vi "Scaled Waveform.vi"(8 "Error In":errorcluster, 11 "Async State Vars In":T1) -> (0 "Error Out":errorcluster, 3 "Async State Vars Out":T1)   [LabVIEW 2015, in "Waveform-Processing-Custom-Device Shared.lvlib" / "Scaled Waveform.lvlib"]
uses:
  Shared/Scaled Waveform/Scaled Waveform.lvlib
  Types/AsyncStateVariables.ctl
  <vilib>/NI Veristand/Custom Device Waveform API/Single Waveform Read (DBL)/Single Waveform Read (DBL).lvclass
  <vilib>/NI Veristand/Custom Device Waveform API/Single Waveform Write (DBL)/Single Waveform Write (DBL).lvclass
  <vilib>/NI Veristand/Custom Device API/Waveform Data Reference.ctl
  <vilib>/NI/NIVS Inline Async API/_Data Access Engine/Data Access Engine/Types/Write.DVR.ctl
  <vilib>/NI/NIVS Inline Async API/_Data Access Engine/Access Type Classes/Write/Write.lvclass
  <vilib>/NI/NIVS Inline Async API/_Data Access Engine/Data Access Engine/Types/Read.DVR.ctl
  <vilib>/NI/NIVS Inline Async API/_Data Access Engine/Access Type Classes/Read/Read.lvclass
  <userlib>/Circular Buffer/Controls/Circular Buffer Operations.ctl
  <userlib>/Circular Buffer/Instance VIs/Circular Buffer(2D DBL).vi
  <userlib>/Circular Buffer/Circular Buffer.lvlib
  <vilib>/NI VeriStand/Custom Device API/Custom Device API.lvlib
  <vilib>/NI/NIVS Inline Async API/_Data Access Engine/Data Access Engine/Data Access Engine.lvclass
  Waveform-Processing-Custom-Device Engine.lvlib
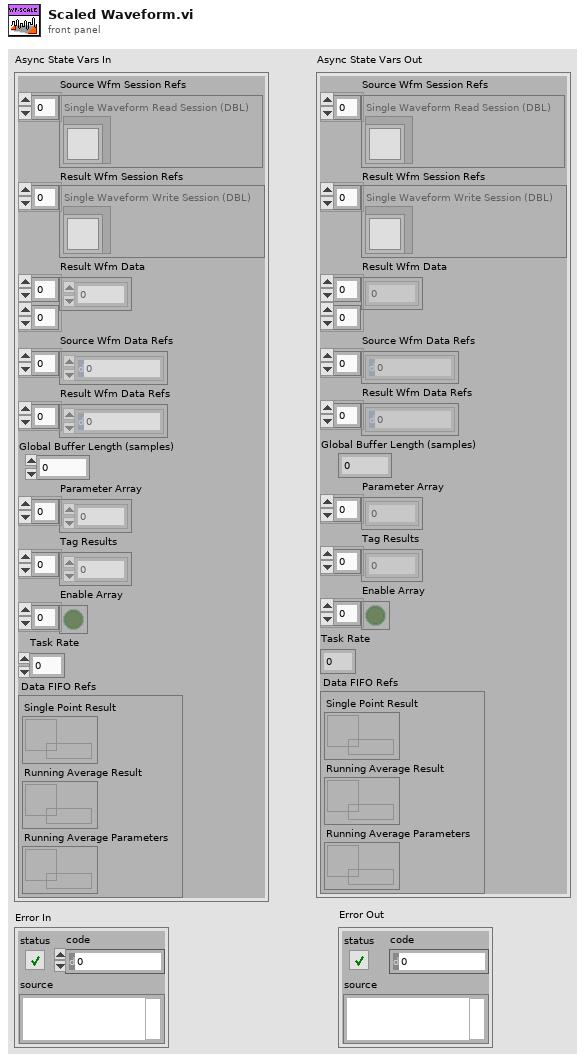
[diagram p1: front panel]
types:
  T1 = typedef "Waveform-Processing-Custom-Device Engine.lvlib/AsyncStateVariables.ctl" = cluster{"Source Wfm Session Refs":refnum<class "Single Waveform Read (DBL).lvclass">[], "Result Wfm Session Refs":refnum<class "Single Waveform Write (DBL).lvclass">[], "Result Wfm Data":dbl[][], "Source Wfm Data Refs":T2[], "Result Wfm Data Refs":T2[], "Global Buffer Length (samples)":dbl, "Parameter Array":dbl[], "Tag Results":dbl[], "Enable Array":bool[], "Task Rate":dbl, "Data FIFO Refs":cluster{"Single Point Result":T3, "Running Average Result":T3, "Running Average Parameters":T4}}
  T2 = typedef "Custom Device API.lvlib/Waveform Data Reference.ctl" = i32
  T3 = typedef "Data Access Engine.lvlib/Data Access Engine.lvclass/Write.DVR.ctl" = refnum<data-value>
  T4 = typedef "Data Access Engine.lvlib/Data Access Engine.lvclass/Read.DVR.ctl" = refnum<data-value>
  T5 = typedef "Circular Buffer.lvlib/Circular Buffer Operations.ctl" = enum16{"Initialize", "Get Backlog", "Write", "Read (continuous)", "Read (most recent)"}
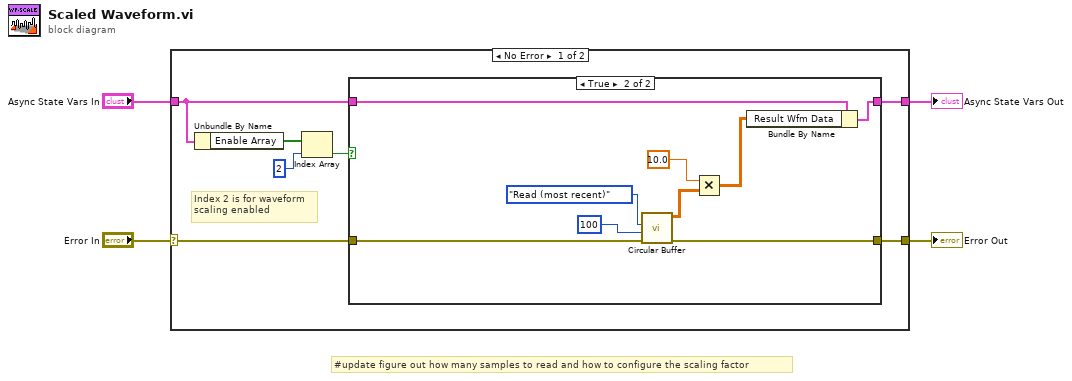
[diagram p0: block diagram]
diagram:
  # "#update figure out how many samples to read and how to configure the scaling factor"
  n1 = case shown="No Error" "Error In" {
    selector: "Error In" -> [w9 w24]
    tunnel: [w5 w24] -> w3
    tunnel: "Async State Vars In" -> [w7 w23]
    tunnel: [w6 w23] -> w1
    frame No Error {
      # "Index 2 is for waveform\nscaling enabled"
      n2 = Unbundle By Name(w7) -> ("Enable Array"=w11:bool[])
      n3 = Index Array(array=w11, index=2) -> (element=w8:bool)
      n4 = case shown="True" w8 {
        tunnel: w9 -> [w12 w22]
        tunnel: w7 -> [w13 w19]
        tunnel: [w13 w18] -> w6
        tunnel: [w12 w14] -> w5
        frame False {
        }
        frame True {
          n5 = call-poly <userlib>:"Circular Buffer.vi"("error in (no error)"=w22, "Read Size"=100, "Operation"=Circular_Buffer_Operations."Read (most recent)") -> ("error out"=w14:errorcluster, "Data Out"=w17:dbl[][])  [unwired: 5 in, 2 out]
          n6 = Multiply(x=10.0 ("element"), y=w17) -> (x*y=w15:dbl[][])
          n7 = Bundle By Name(cluster=w19, "Result Wfm Data"=w15) -> (w18:T1)
        }
      }
    }
    frame Error {
    }
  }
  "Async State Vars Out" <- w1
  "Error Out" <- w3
